vi "Save Plotted Data File Rows.vi"(5 "Results Folders":path[](array[path])) -> ()   [LabVIEW 2022 SP3]
uses:
  1f57b876-2685-48c4-9434-55530a3eb207.vi
  Anemometry/Anemometry Sub Vis/Data_plotting_vis/Results_plotter_Global.vi
  <vilib>/Comparison/Less/Less Functor/Less Functor.lvclass
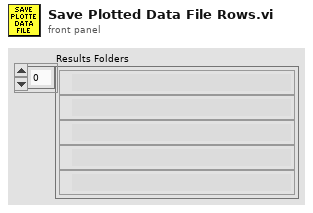
[diagram p1: front panel]
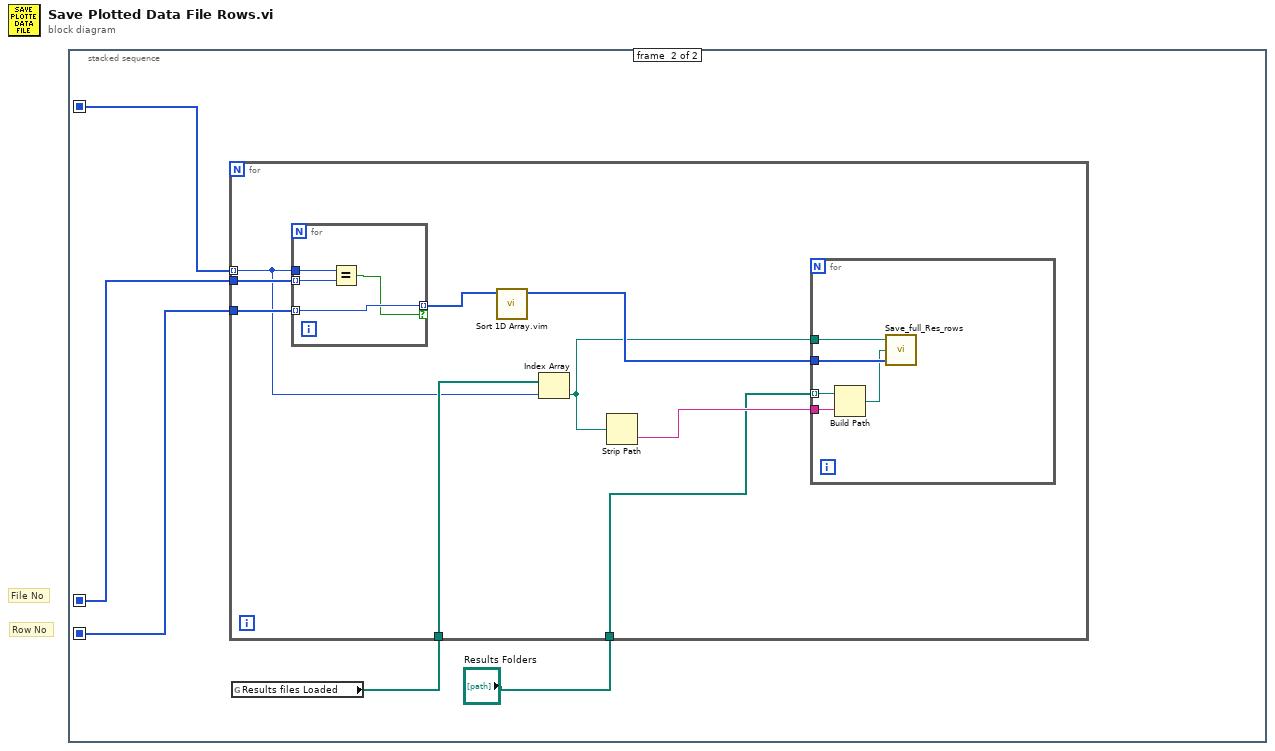
[diagram p0: block diagram]
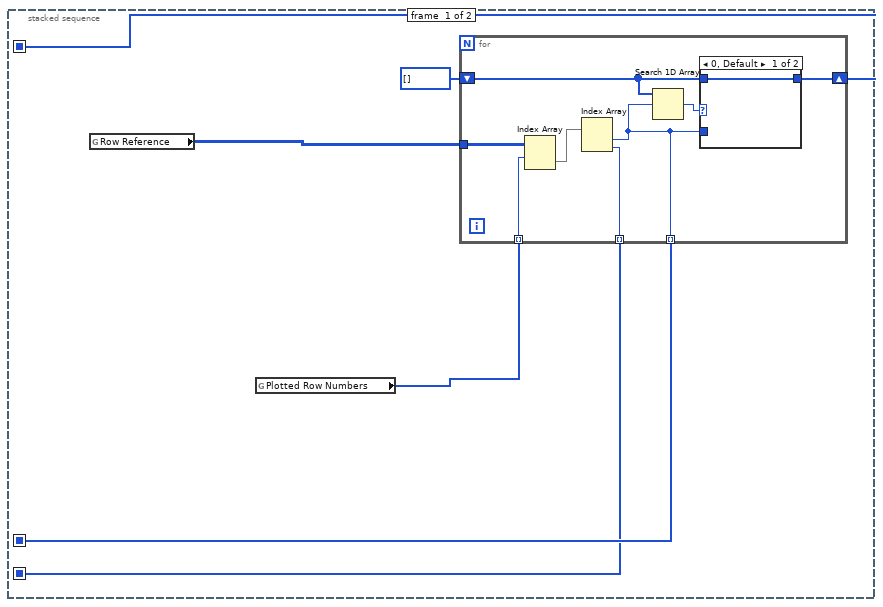
[diagram p2: hidden frame]
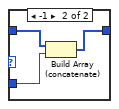
[diagram p3: hidden frame]
diagram:
  # "Row No"
  # "File No"
  n1 = stacked-sequence {
    seq-local: [w2 _] -> [_ w21]
    seq-local: [w4 _] -> [_ w22]
    seq-local: [w3 _] -> [_ w23]
    frame #0 {
      n2 = global read "Results_plotter_Global.vi" "Row Reference"() -> (w6:i32[][])
      n3 = global read "Results_plotter_Global.vi" "Plotted Row Numbers"() -> (w1:i32[])
      n4 = for {
        tunnel: w1 -> [w14] mode=indexing
        tunnel: w6 -> [w13]
        shift-right: [w9] -> w3
        shift-left: i32[] [] -> [w10]
        tunnel: [w8] -> w4 mode=indexing
        tunnel: [w7] -> w2 mode=indexing
        n5 = Index Array(array=w13, index (row)=w14) -> (element=w12:i32[])  [unwired: 1 in]
        n6 = Index Array(array=w12) -> (element #1=w8:i32, element #2=w7:i32)  [unwired: 2 in]
        n7 = Search 1D Array(1D array=w10, element=w8) -> (index of element=w11:i32)  [unwired: 1 out]
        n8 = case shown="0, Default" w11 {
          tunnel: w10 -> [w15 w18]
          tunnel: w8 -> [_ w17]
          tunnel: [w15 w16] -> w9
          frame 0, Default {
          }
          frame -1 {
            n9 = Build Array (concatenate)(w18, w17) -> (w16:i32[])
          }
        }
      }
    }
    frame #1 {
      n10 = global read "Results_plotter_Global.vi" "Results files Loaded"() -> (w20:path[])
      n11 = for {
        tunnel: w23 -> [w27] mode=indexing
        tunnel: w22 -> [w32]
        tunnel: w21 -> [w31]
        tunnel: w20 -> [w28]
        tunnel: "Results Folders" -> [w24]
        n12 = for {
          tunnel: w27 -> [w41]
          tunnel: w32 -> [w40] mode=indexing
          tunnel: [w39] -> w30 mode=indexing if=w38
          tunnel: w31 -> [w39] mode=indexing
          n13 = Equal?(x=w41, y=w40) -> (x = y?=w38:bool)
        }
        n14 = call "Sort 1D Array.vim"("unsorted array"=w30) -> ("sorted array"=w29:i32[])  [unwired: 10 in]
        n15 = Index Array(array=w28, index=w27) -> (element=w26:path)
        n16 = Strip Path(path=w26) -> (name=w25:string)  [unwired: 1 out]
        n17 = for {
          tunnel: w29 -> [w37]
          tunnel: w26 -> [w36]
          tunnel: w25 -> [w35]
          tunnel: w24 -> [w33] mode=indexing
          n18 = Build Path(base path=w33, name or relative path=w35) -> (appended path=w34:path)
          n19 = call "Save_full_Res_rows.vi"("Selected Rows"=w37, "Filename to write"=w34, "Filename Orig"=w36) -> ()  [unwired: 2 out]
        }
      }
    }
  }
